vi "Post-select init.vi"(7 "Init DIH params?":bool, 9 "Input event data":T2, 10 "Inspection.Image details_init":T1(array[cluster])) -> (1 "Number of racks":u8, 2 "Inspection.Image details_init":T1(array[cluster]))   [LabVIEW 2019, in "ZenGage v3.0 UI.lvclass"]
uses:
  ZenGage v3.0 UI.lvclass
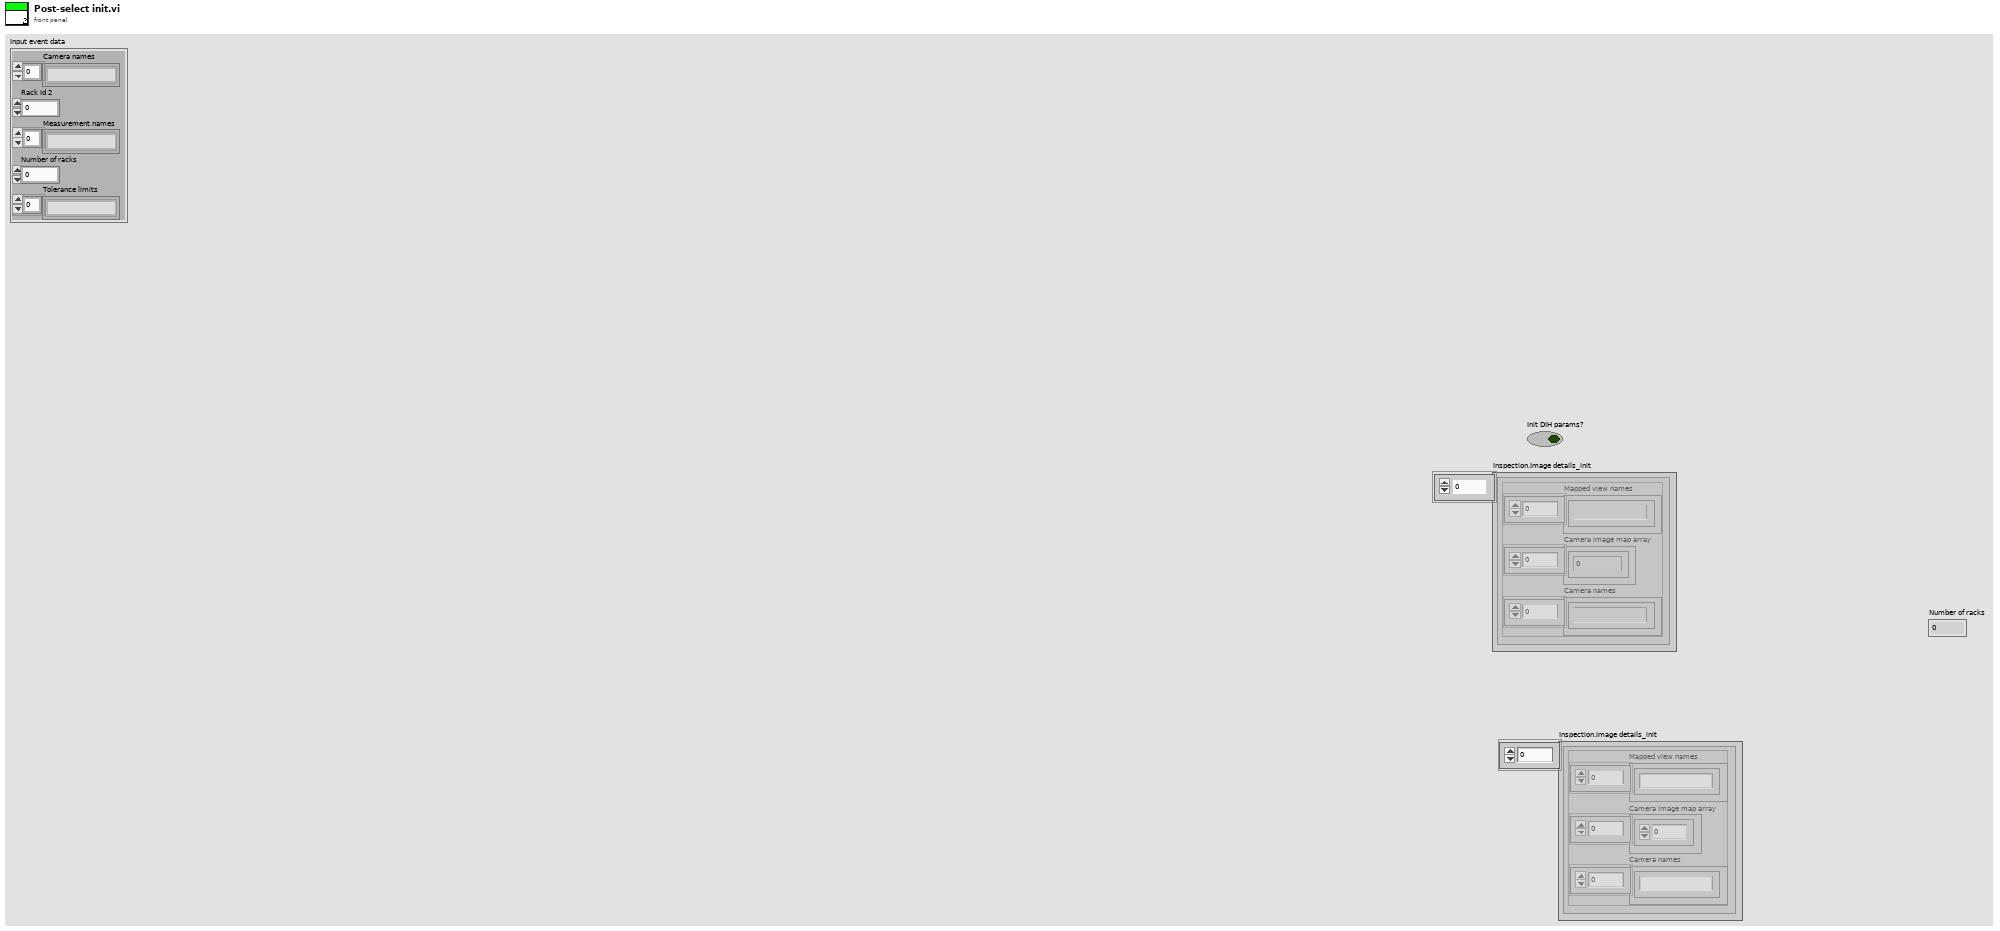
[diagram p1: front panel]
types:
  T1 = cluster{"Mapped view names":string[], "Camera image map array":i32[], "Camera names":string[]}[]
  T2 = cluster{"Camera names":string[], "Rack Id 2":u8, "Measurement names":string[], "Number of racks":u8, "Tolerance limits":string[]}
  T3 = cluster{"Mapped view names":string[], "Camera image map array":i32[], "Camera names":string[]}
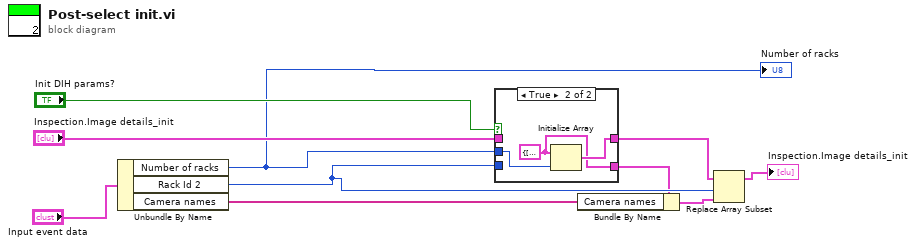
[diagram p0: block diagram]
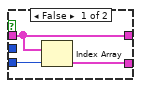
[diagram p2: hidden frame]
diagram:
  n1 = Unbundle By Name("Input event data") -> ("Number of racks"=w1:u8, "Rack Id 2"=w6:u8, "Camera names"=w10:string[])
  "Number of racks" <- w1
  n2 = case shown="True" "Init DIH params?" {
    tunnel: w6 -> [w13 _]
    tunnel: "Inspection.Image details_init" -> [w11 _]
    tunnel: w1 -> [_ w16]
    tunnel: [w12 w14] -> w3
    tunnel: [w11 w15] -> w2
    frame False {
      n3 = Index Array(array=w11, index=w13) -> (element=w12:T3)
    }
    frame True {
      w14 = T3 {"Mapped view names"=[], "Camera image map array"=[], "Camera names"=[]} ("Rack based image\ndetails")
      n4 = Initialize Array(w14, w16) -> (w15:T1)
    }
  }
  n5 = Bundle By Name(cluster=w3, "Camera names"=w10) -> (w9:T3)
  n6 = Replace Array Subset(array=w2, new element=w9, index=w6) -> (→"Inspection.Image details_init":T1)
